vi "Tank_Mecanum_Drive_Cartesian.vi"(6 "Left X":dbl, 8 "error in (no error)":errorcluster, 9 "Left Y":dbl, 10 "Right Y":dbl, 11 "RobotDriveDevRef":T1={"DevStatus"={"status"=FALSE, "code"=0, "source"=""}, "Motors[]"=[], "Square Inputs"=FALSE, "Max Output"=1.0, "Isochronous"=FALSE}) -> (0 "error out":errorcluster, 2 "Motor Values":dbl[](array[numeric]), 3 "RobotDriveDevRef":T1={"DevStatus"={"status"=FALSE, "code"=0, "source"=""}, "Motors[]"=[], "Square Inputs"=FALSE, "Max Output"=1.0, "Isochronous"=FALSE})   [LabVIEW 2013]
doc: "Configures the motors for holonomic driving. Holonomic driving allows you to move the robot in any direction without first rotating or maneuvering the robot.\n\nThis VI requires the robot to have either four omni-directional wheels and four motors mounted at 45 degree angles in the four corners of a square frame or to have four mecanum wheels driven by four motors.\n\nThe control input is intended to be connected directly to the X, Y, and Z axes of a joystick. The Y axis is inverted for you.\n\nThis software is licensed. Open the labview\\readme\\WPI Robotics Library Open Source License.txt file for more information."
uses:
  <vilib>/Rock Robotics/WPI/RobotDrive/WPI_RobotDriveDevRef.ctl
  <vilib>/Rock Robotics/WPI/MotorControl/WPI_MotorControlDeviceRef.ctl
  <vilib>/Rock Robotics/SystemInterfaces/Typedef/FPGA_TypedefDigitalModule.ctl
  <vilib>/Rock Robotics/SystemInterfaces/DIO/FPGA_DIOPWMChannel.ctl
  <vilib>/Rock Robotics/WPI/PWM/WPI_PWMDeadband.ctl
  <vilib>/Rock Robotics/WPI/CAN/Jaguar/SubVIs/WPI_CANJaguar_ControlMode.ctl
  <vilib>/Rock Robotics/WPI/PWM/WPI_PWMTransform_ConPane.ctl
  <vilib>/Rock Robotics/SystemInterfaces/NetworkCommunication/NetComm_UsageReport_ResourceType.ctl
  <vilib>/Rock Robotics/WPI/RobotDrive/WPI_RobotDriveMotorSelectorEnum.ctl
  <vilib>/Rock Robotics/WPI/RobotDrive/WPI_RobotDriveSafetyCheck.vi
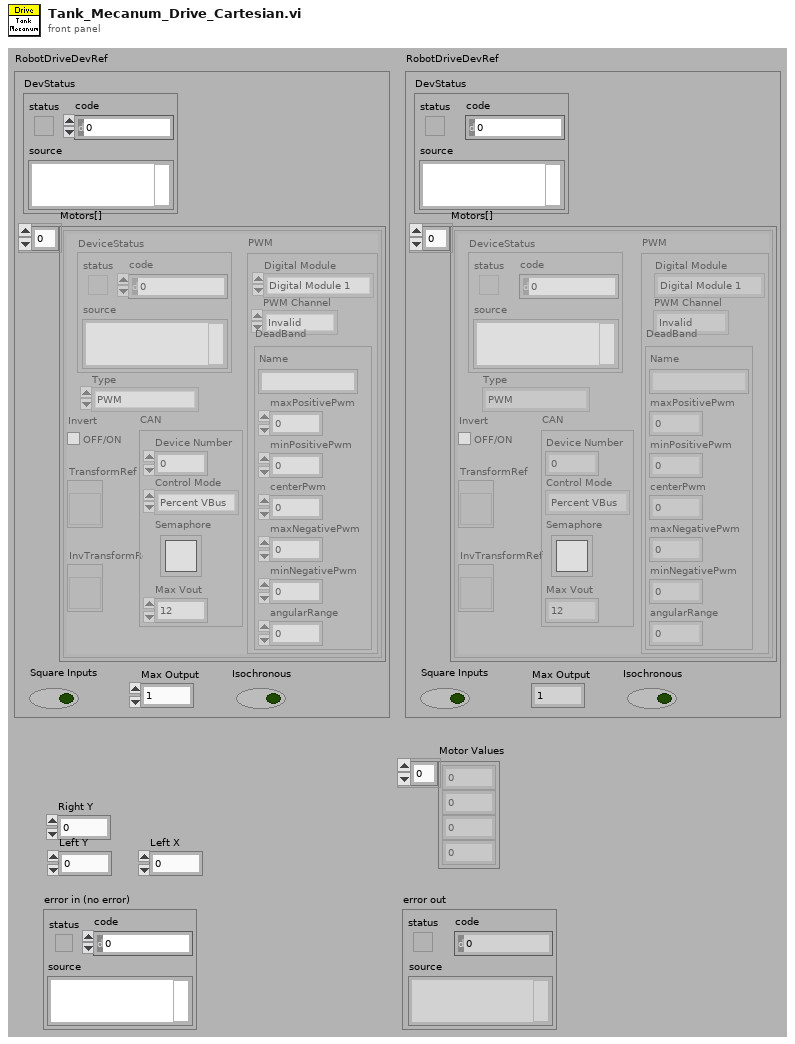
[diagram p1: front panel]
types:
  T1 = typedef "WPI_RobotDriveDevRef.ctl" = cluster{"DevStatus":errorcluster, "Motors[]":T2[], "Square Inputs":bool, "Max Output":dbl, "Isochronous":bool}
  T2 = typedef "WPI_MotorControlDeviceRef.ctl" = cluster{"DeviceStatus":errorcluster, "Type":enum16{"PWM", "CAN"}, "PWM":cluster{"Digital Module":T3, "PWM Channel":T4, "DeadBand":T5}, "CAN":cluster{"Device Number":u8, "Control Mode":T6, "Semaphore":T7, "Max Vout":dbl}, "Invert":bool, "TransformRef":T8, "InvTransformRef":T8}
  T3 = typedef "FPGA_TypedefDigitalModule.ctl" = enum16{"Digital Module 1", "Digital Module 2"}
  T4 = typedef "FPGA_DIOPWMChannel.ctl" = enum8{"PWM 1", "PWM 2", "PWM 3", "PWM 4", "PWM 5", "PWM 6", "PWM 7", "PWM 8", "PWM 9", "PWM 10", "Invalid"}
  T5 = typedef "WPI_PWMDeadband.ctl" = cluster{"Name":string, "maxPositivePwm":i32, "minPositivePwm":i32, "centerPwm":i32, "maxNegativePwm":i32, "minNegativePwm":i32, "angularRange":u16}
  T6 = typedef "WPI_CANJaguar_ControlMode.ctl" = enum8{"Percent VBus", "Current", "Speed", "Position", "Voltage"}
  T7 = typedef "Semaphore RefNum" = refnum<k1>
  T8 = typedef "WPI_PWMTransform_ConPane.ctl" = refnum<vi>
  T9 = typedef "NetComm_UsageReport_ResourceType.ctl" = enum8{"Controller", "Module", "Language", "CANPlugin", "Accelerometer", "ADXL345", "AnalogChannel", "AnalogTrigger", "AnalogTriggerOutput", "CANJaguar", "Compressor", "Counter", "Dashboard", "DigitalInput", "DigitalOutput", "DriverStationCIO", "DriverStationEIO", "DriverStationLCD", "Encoder", "GearTooth", "Gyro", "I2C", "Framework", "Jaguar", "Joystick", "Kinect", "KinectStick", "PIDController", "Preferences", "PWM", "Relay", "RobotDrive", "SerialPort", "Servo", "Solenoid", "SPI", "Task", "Ultrasonic", "Victor", "Button", "Command", "AxisCamera", "PCVideoServer", "SmartDashboard", "Talon", "HiTechnicColorSensor", "HiTechnicAccel", "HiTechnicCompass", "SRF08"}
  T10 = typedef "WPI_RobotDriveMotorSelectorEnum.ctl" = enum16{"Rear Left Motor", "Rear Right Motor", "Front Left Motor", "Front Right Motor"}
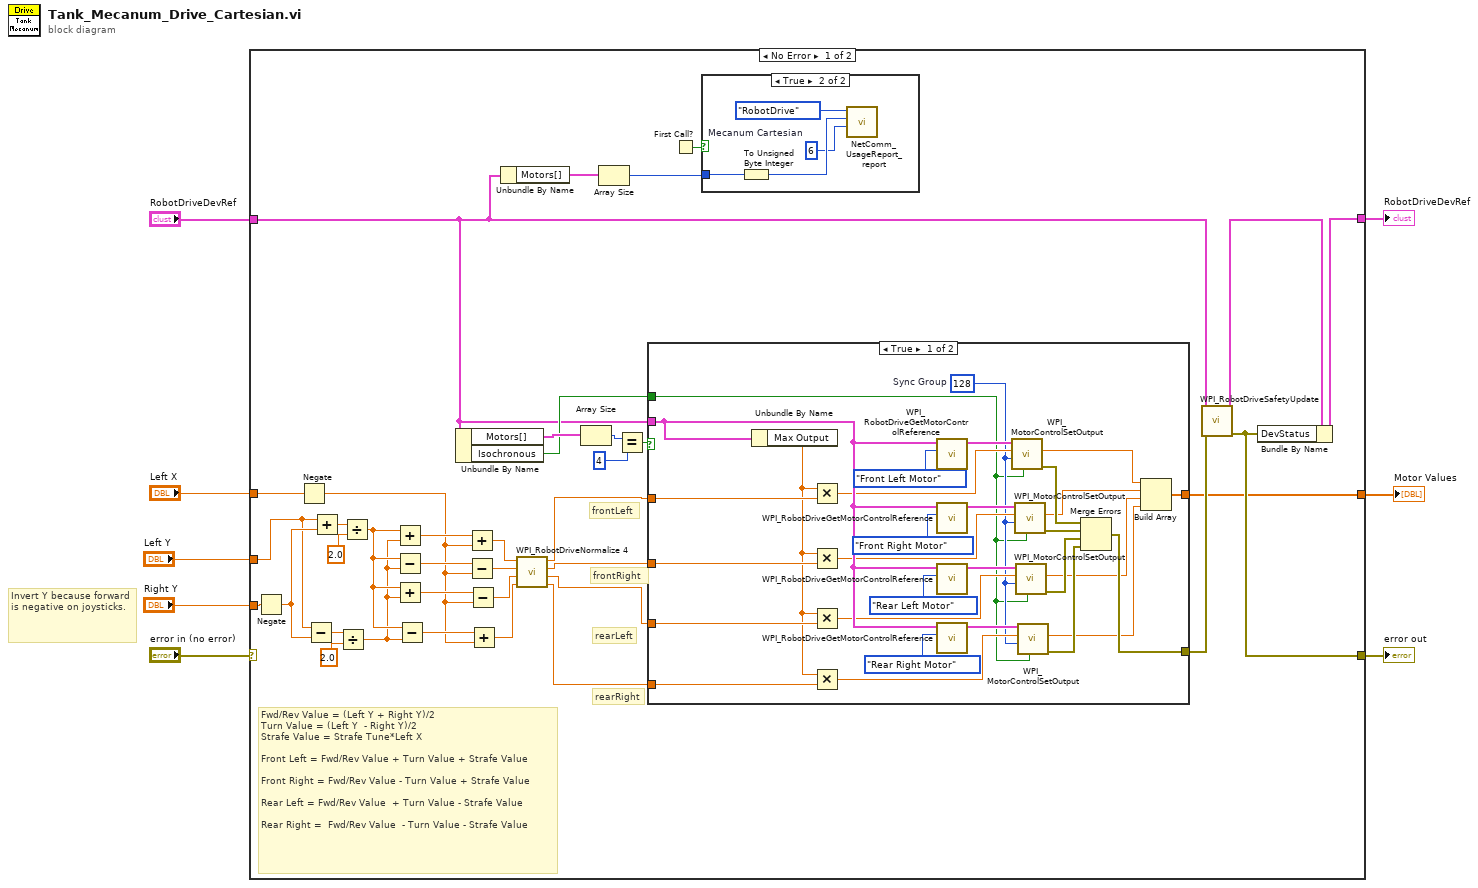
[diagram p0: block diagram]
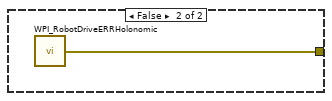
[diagram p3: hidden frame]
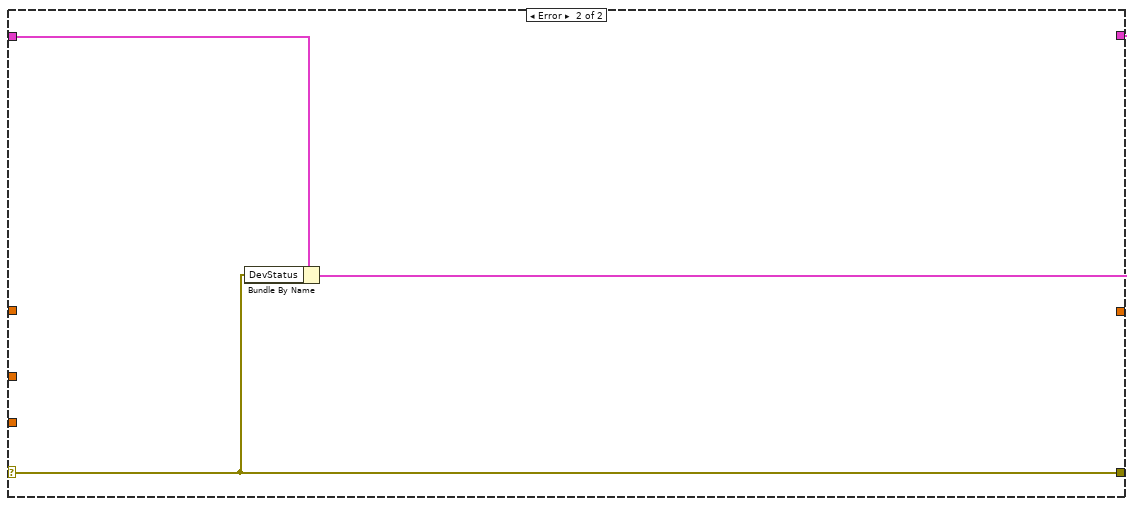
[diagram p4: hidden frame]
diagram:
  # "Invert Y because forward is negative on joysticks."
  n1 = case shown="No Error" "error in (no error)" {
    selector: "error in (no error)" -> [_ w81]
    tunnel: "Left Y" -> [w10 _]
    tunnel: "Right Y" -> [w17 _]
    tunnel: "RobotDriveDevRef" -> [w29 w83]
    tunnel: [w42 w82] -> w4
    tunnel: [w35 w81] -> w3
    tunnel: "Left X" -> [w27 _]
    tunnel: [w28 _] -> w1
    frame No Error {
      # "Fwd/Rev Value = (Left Y + Right Y)/2\nTurn Value = (Left Y  - Right Y)/2 \nStrafe Value = Strafe Tune*Left X\n\nFront Left = Fwd/Rev Value + Turn Value + Strafe Value\n\nFront Right = Fwd/Rev Value - Turn Value + Strafe Value\n\nRear Left = Fwd/Rev Value  + Turn Value - Strafe Value\n\nRear Right =  Fwd/Rev Value  - Turn Value - Strafe Value"
      # "rearLeft"
      # "frontRight"
      # "rearRight"
      # "frontLeft"
      n2 = Negate(x=w17) -> (-x=w16:dbl)
      n3 = Negate(x=w27) -> (-x=w11:dbl)
      n4 = Subtract(x=w10, y=w16) -> (x-y=w21:dbl)
      n5 = Add(x=w10, y=w16) -> (x+y=w22:dbl)
      n6 = Divide(x=w21, y=2.0) -> (x/y=w12:dbl)
      n7 = Divide(x=w22, y=2.0) -> (x/y=w18:dbl)
      n8 = Add(x=w18, y=w12) -> (x+y=w13:dbl)
      n9 = Subtract(x=w18, y=w12) -> (x-y=w14:dbl)
      n10 = Add(x=w18, y=w12) -> (x+y=w15:dbl)
      n11 = Subtract(x=w18, y=w12) -> (x-y=w19:dbl)
      n12 = Unbundle By Name(w29) -> ("Motors[]"=w34:T2[], "Isochronous"=w33:bool)
      n13 = Add(x=w13, y=w11) -> (x+y=w26:dbl)
      n14 = Subtract(x=w14, y=w11) -> (x-y=w25:dbl)
      n15 = Subtract(x=w15, y=w11) -> (x-y=w24:dbl)
      n16 = Add(x=w19, y=w11) -> (x+y=w23:dbl)
      n17 = Unbundle By Name(w29) -> ("Motors[]"=w31:T2[])
      n18 = call <vilib>:"WPI_RobotDriveNormalize 4.vi"("D"=w23, "C"=w24, "B"=w25, "A"=w26) -> ("D'"=w39:dbl, "C'"=w38:dbl, "B'"=w40:dbl, "A'"=w41:dbl)
      n19 = Array Size(array=w34) -> (size(s)=w45:i32)
      n20 = Array Size(array=w31) -> (size(s)=w30:i32)
      n21 = Equal?(x=w45, y=4) -> (x = y?=w43:bool)
      n22 = case shown="True" w43 {
        tunnel: w41 -> [w79 _]
        tunnel: w40 -> [w78 _]
        tunnel: w29 -> [w67 _]
        tunnel: [w57 w80] -> w37
        tunnel: w38 -> [w73 _]
        tunnel: w39 -> [w72 _]
        tunnel: w33 -> [w55 _]
        tunnel: [w53 _] -> w28
        frame True {
          w56 = u8 128  # Sync Group
          n23 = Unbundle By Name(w67) -> ("Max Output"=w62:dbl)
          n24 = Multiply(x=w62, y=w79) -> (x*y=w66:dbl)
          n25 = Multiply(x=w62, y=w78) -> (x*y=w65:dbl)
          n26 = Multiply(x=w62, y=w73) -> (x*y=w64:dbl)
          n27 = Multiply(x=w62, y=w72) -> (x*y=w63:dbl)
          n28 = call <vilib>:"WPI_RobotDriveGetMotorControlReference.vi"("MotorIndex"=WPI_RobotDriveMotorSelectorEnum."Front Left Motor", "RobotDriveDevRef"=w67) -> ("MotorControlDeviceRef"=w77:T2)  [unwired: 9 out]
          n29 = call <vilib>:"WPI_RobotDriveGetMotorControlReference.vi"("MotorIndex"=WPI_RobotDriveMotorSelectorEnum."Front Right Motor", "RobotDriveDevRef"=w67) -> ("MotorControlDeviceRef"=w75:T2)  [unwired: 9 out]
          n30 = call <vilib>:"WPI_RobotDriveGetMotorControlReference.vi"("MotorIndex"=WPI_RobotDriveMotorSelectorEnum."Rear Left Motor", "RobotDriveDevRef"=w67) -> ("MotorControlDeviceRef"=w76:T2)  [unwired: 9 out]
          n31 = call <vilib>:"WPI_RobotDriveGetMotorControlReference.vi"("MotorIndex"=WPI_RobotDriveMotorSelectorEnum."Rear Right Motor", "RobotDriveDevRef"=w67) -> ("MotorControlDeviceRef"=w74:T2)  [unwired: 9 out]
          n32 = call <vilib>:"WPI_MotorControlSetOutput.vi"("Isochronous"=w55, "Sync Group"=w56, "Output"=w66, "MotorControlDevRef"=w77) -> ("error out"=w58:errorcluster, "Motor Output"=w54:dbl)  [unwired: 1 in, 5 out]
          n33 = call <vilib>:"WPI_MotorControlSetOutput.vi"("Isochronous"=w55, "Sync Group"=w56, "Output"=w65, "MotorControlDevRef"=w75) -> ("error out"=w59:errorcluster, "Motor Output"=w52:dbl)  [unwired: 1 in, 5 out]
          n34 = call <vilib>:"WPI_MotorControlSetOutput.vi"("Isochronous"=w55, "Sync Group"=w56, "Output"=w64, "MotorControlDevRef"=w76) -> ("error out"=w60:errorcluster, "Motor Output"=w51:dbl)  [unwired: 1 in, 5 out]
          n35 = call <vilib>:"WPI_MotorControlSetOutput.vi"("Isochronous"=w55, "Sync Group"=w56, "Output"=w63, "MotorControlDevRef"=w74) -> ("error out"=w61:errorcluster, "Motor Output"=w50:dbl)  [unwired: 1 in, 5 out]
          n36 = Merge Errors(w58, w59, w60, w61) -> (w57:errorcluster)
          n37 = Build Array(w54, w52, w51, w50) -> (w53:dbl[])
        }
        frame False {
          n38 = call <vilib>:"WPI_RobotDriveERRHolonomic.vi"() -> ("error out"=w80:errorcluster)
        }
      }
      n39 = First Call?() -> (First Call?: T/F=w32:bool)
      n40 = case shown="True" w32 {
        tunnel: w30 -> [_ w48]
        frame False {
        }
        frame True {
          w46 = u8 6  # Mecanum Cartesian
          n41 = To Unsigned Byte Integer(number=w48) -> (unsigned 8bit integer=w47:u8)
          n42 = call <vilib>:"NetComm_UsageReport_report.vi"("Context"=w46, "Instance Number"=w47, "Resource Type"=NetComm_UsageReport_ResourceType."RobotDrive") -> ()  [unwired: 9 in]
        }
      }
      n43 = call <vilib>:"WPI_RobotDriveSafetyUpdate.vi"("error in (no error)"=w37, "RobotDriveDevRef"=w29) -> ("error out"=w35:errorcluster, "RobotDriveDevRef"=w36:T1)  [unwired: 8 out]
      n44 = Bundle By Name(cluster=w36, "DevStatus"=w35) -> (w42:T1)
    }
    frame Error {
      n45 = Bundle By Name(cluster=w83, "DevStatus"=w81) -> (w82:T1)
    }
  }
  "error out" <- w3
  "RobotDriveDevRef" <- w4
  "Motor Values" <- w1
